vi "Error Handler Queue.vi"(8 "error in (no error)":errorcluster, 11 "VI Refnum":refnum<vi>) -> (0 "error out":errorcluster)   [LabVIEW 2018, in "Mensajes.lvlib"]
uses:
  Mensajes.lvlib
  Controles/FGV Opciones.ctl
  Controles/Lista Modulos.ctl
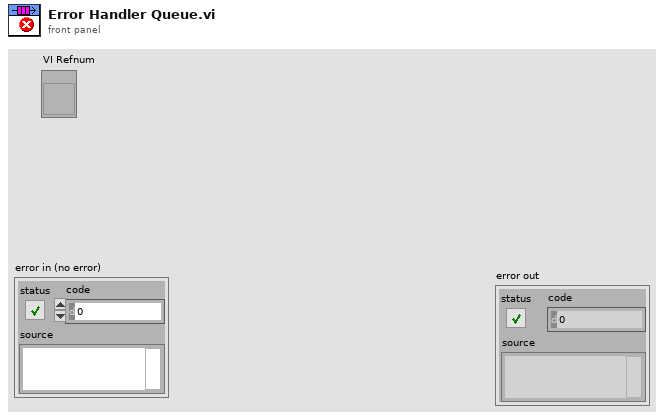
[diagram p1: front panel]
types:
  T1 = typedef "Lista Modulos.ctl" = enum16{"Error", "UI", "Controler", "Config", "Database"}
  T2 = typedef "FGV Opciones.ctl" = enum16{"Get", "Create", "Destroy"}
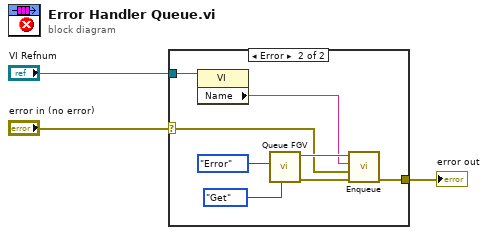
[diagram p0: block diagram]
diagram:
  n1 = case shown="Error" "error in (no error)" {
    selector: "error in (no error)" -> [w4 w7]
    tunnel: [w4 w8] -> w3
    tunnel: "VI Refnum" -> [_ w6]
    frame No Error {
    }
    frame Error {
      n2 = property class="VI"(reference=w6) -> ("Name"=w5:string)  [unwired: 1 in, 2 out]
      n3 = call "Queue FGV.vi"("Enum"=FGV_Opciones."Get", "Modulo a obtener"=Lista_Modulos."Error") -> ("error out"=w9:errorcluster, "Queue Ref"=w10:refnum<queue>)  [unwired: 8 in]
      n4 = call "Enqueue.vi"("error in (no error)"=w9, "Dato"=w7, "Mensaje"=w5, "Queue in"=w10) -> ("error out"=w8:errorcluster)  [unwired: 7 in]
    }
  }
  "error out" <- w3
